vi "Main.vi"(8 "error in":errorcluster, 11 "Modbus PLC in":refnum<class "Modbus PLC.lvclass">) -> (0 "error out":errorcluster, 3 "Modbus PLC out":refnum<class "Modbus PLC.lvclass">)   [LabVIEW 2023, in "Modbus PLC.lvlib" / "Modbus PLC.lvclass"]
doc: "The <b>Queued Message Handler</b> of the Worker that owns this VI."
uses:
  Modbus PLC.lvclass
  J:/Work/Cortech/KTM 1001/Workers Hardware/Workers/Base Classes/Base Hardware/Base Hardware.lvclass
  C:/Program Files/National Instruments/LabVIEW 2023/vi.lib/addons/_Workers/Library/Classes/Worker/Worker.lvclass
  Commands.ctl
  Data.ctl
  Settings.ctl
  Workers Hardware/Workers/Base Classes/Base Hardware/rqp_Update Internal Data.ctl
  rqp_Write Rotate.ctl
  rqp_Write Termex.ctl
  rqp_Write Mix.ctl
  rqp_Write Numeric Parameter.ctl
  <vilib>/Utility/error.llb/Error Cluster From Error Code.vi
  <vilib>/ErrorRing/Error Ring.xnode
  <vilib>/addons/_Workers/Library/Classes/Message Queue/Message Queue.lvclass
  Workers Hardware/Workers/Base Classes/Base Hardware/Base Hardware.lvclass
panel:
  in  "Settings":T1={"IP Address"="localhost", "Port"=502}
  in  "Connect Btn":bool
  out "IND":T2 {"Rotate_IND" items=["стоп", "Качалка Режим Авто", "Качалка Режим Ручной"]; "Termex_IND" items=["Термостат старт"=1, "Термостат стоп"=0]; "Mix_IND" items=["Мешалка движение вперёд"=1, "Мешалка движение назад"=2, "Мешалка стоп"=0]}
  in  "CMD":T3 {"Mix_CMD" items=["Мешалка движение вперёд"=1, "Мешалка движение назад"=2, "Мешалка стоп"=9]; "Termex_CMD" items=["Термостат старт"=1, "Термостат стоп"=9]; "Rotate_CMD" items=["Качалка Дом"=1, "Качалка Режим Авто - Старт"=2, "Качалка Режим Ручной - Старт"=3, "Качалка Стоп"=9]}
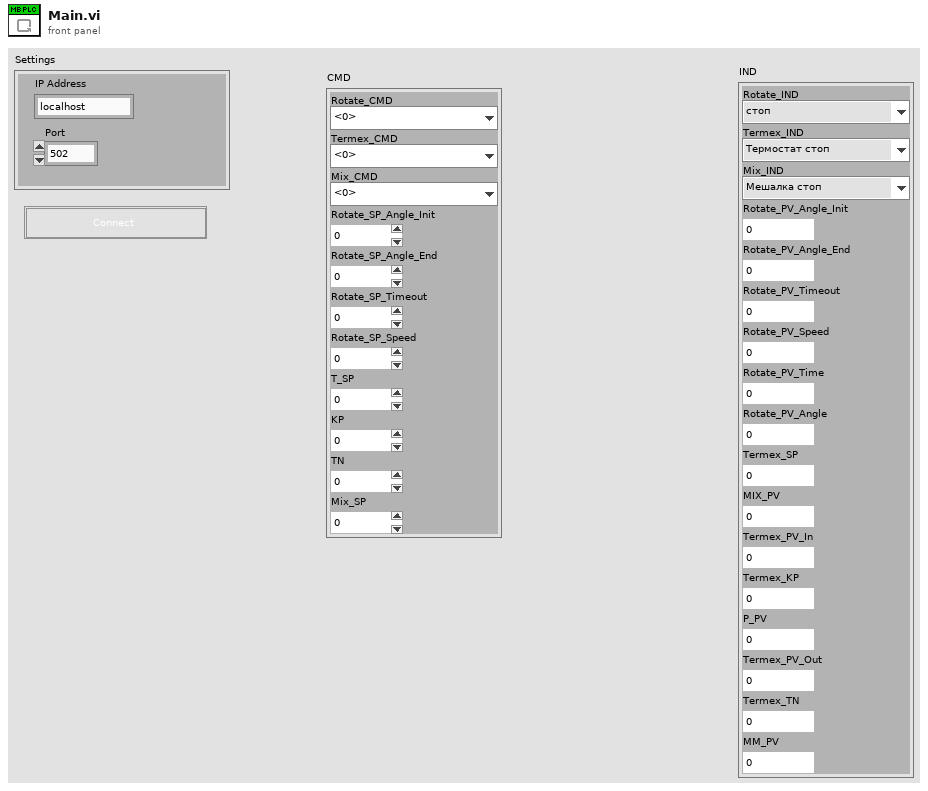
[diagram p1: front panel]
types:
  T1 = typedef "Modbus PLC.lvlib/Modbus PLC.lvclass/Settings.ctl" = cluster{"IP Address":string, "Port":u16}
  T2 = typedef "Modbus PLC.lvlib/Modbus PLC.lvclass/Data.ctl" = cluster{"Rotate_IND":u16, "Termex_IND":u16, "Mix_IND":u16, "Rotate_PV_Angle_Init":u16, "Rotate_PV_Angle_End":u16, "Rotate_PV_Timeout":u16, "Rotate_PV_Speed":u16, "Rotate_PV_Time":u16, "Rotate_PV_Angle":u16, "Termex_SP":sgl, "MIX_PV":u16, "Termex_PV_In":sgl, "Termex_KP":sgl, "P_PV":sgl, "Termex_PV_Out":sgl, "Termex_TN":sgl, "MM_PV":sgl}
  T3 = typedef "Modbus PLC.lvlib/Modbus PLC.lvclass/Commands.ctl" = cluster{"Rotate_CMD":u16, "Termex_CMD":u16, "Mix_CMD":u16, "Rotate_SP_Angle_Init":u16, "Rotate_SP_Angle_End":u16, "Rotate_SP_Timeout":u16, "Rotate_SP_Speed":u16, "T_SP":sgl, "KP":sgl, "TN":sgl, "Mix_SP":u16}
  T4 = typedef "Abstract Hardware.lvlib/Base Hardware.lvclass/rqp_Update Internal Data.ctl" = variant
  T5 = typedef "Modbus PLC.lvlib/Modbus PLC.lvclass/rqp_Write Numeric Parameter.ctl" = cluster{"Parameter":string, "Data":variant}
  T6 = typedef "Modbus PLC.lvlib/Modbus PLC.lvclass/rqp_Write Rotate.ctl" = u16
  T7 = typedef "Modbus PLC.lvlib/Modbus PLC.lvclass/rqp_Write Termex.ctl" = u16
  T8 = typedef "Modbus PLC.lvlib/Modbus PLC.lvclass/rqp_Write Mix.ctl" = u16
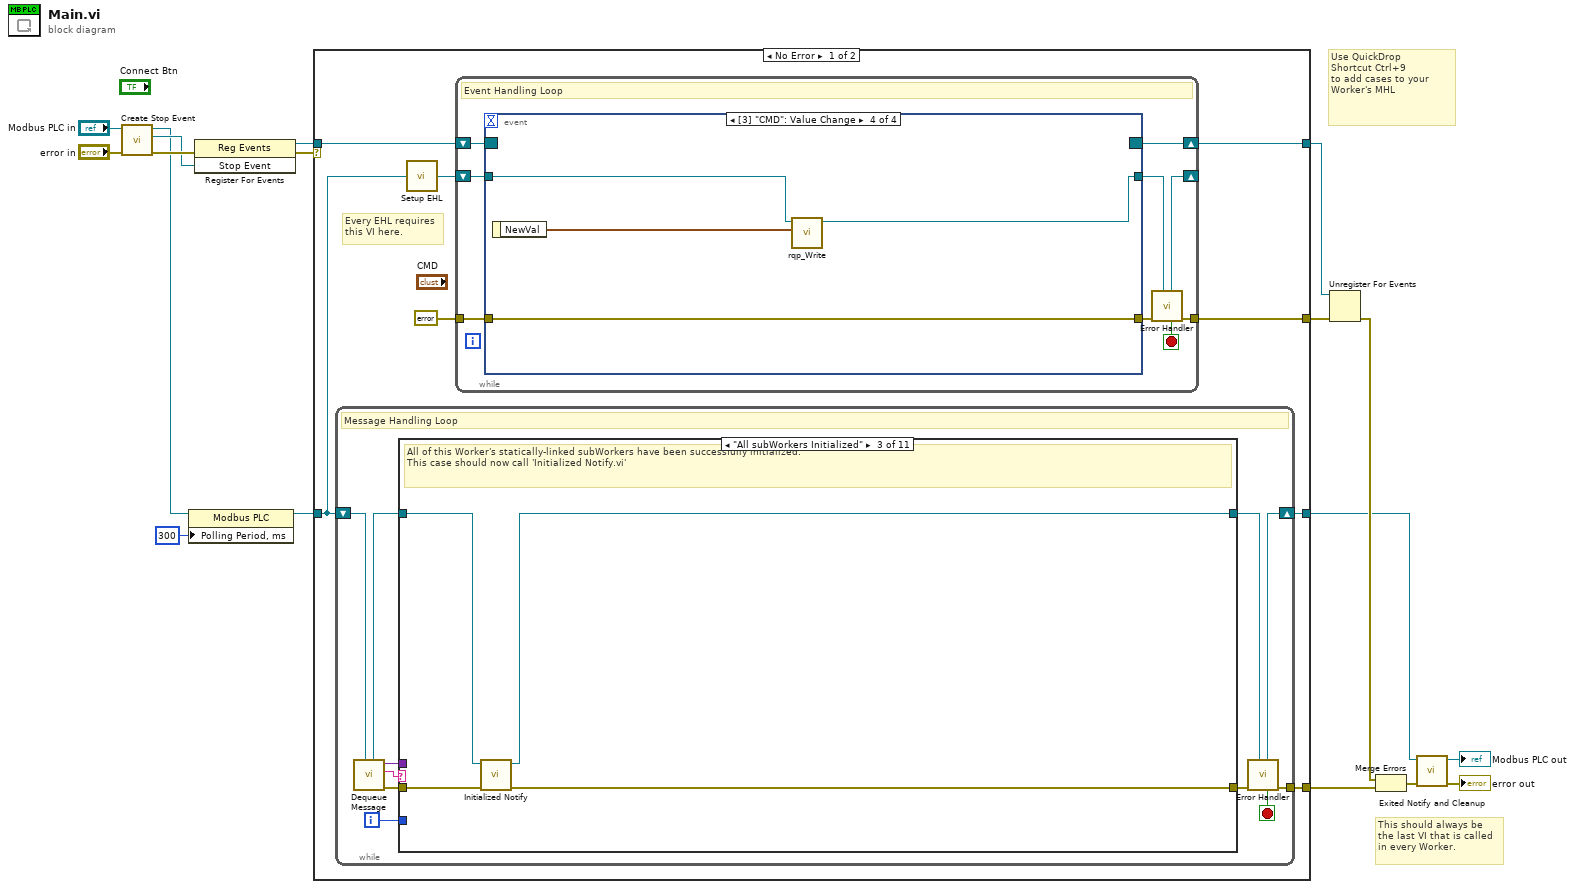
[diagram p0: block diagram]
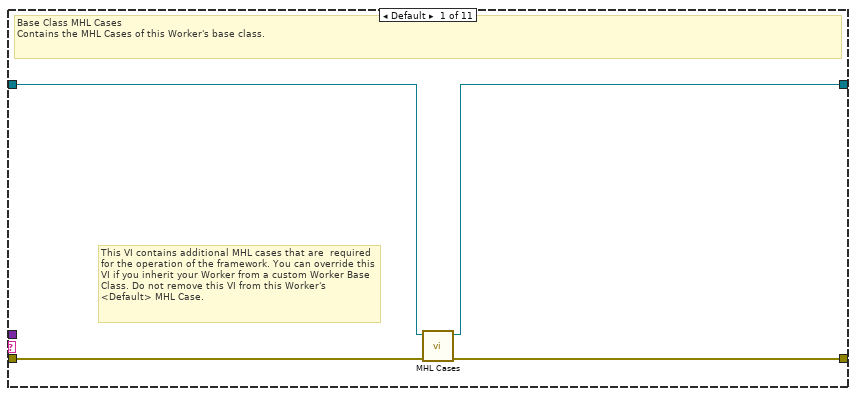
[diagram p2: hidden frame]
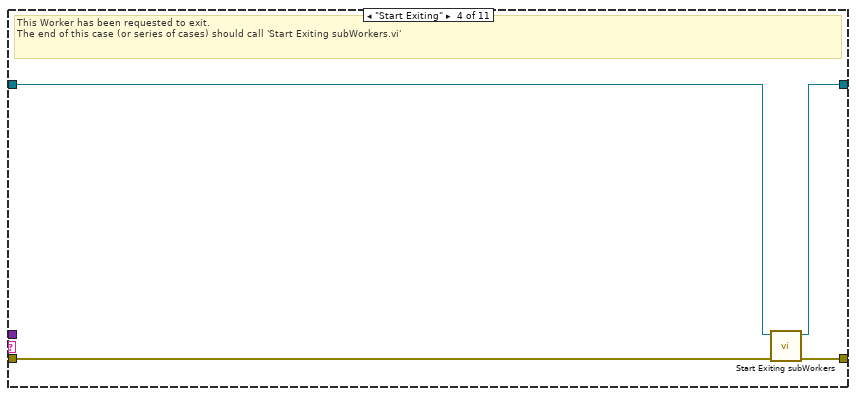
[diagram p4: hidden frame]
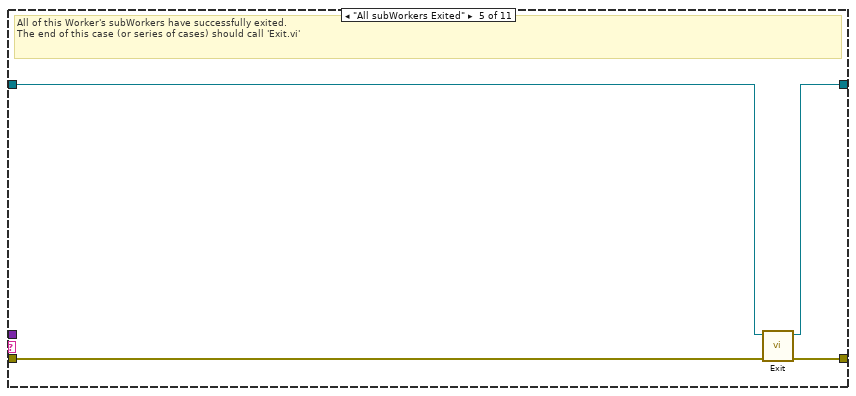
[diagram p5: hidden frame]
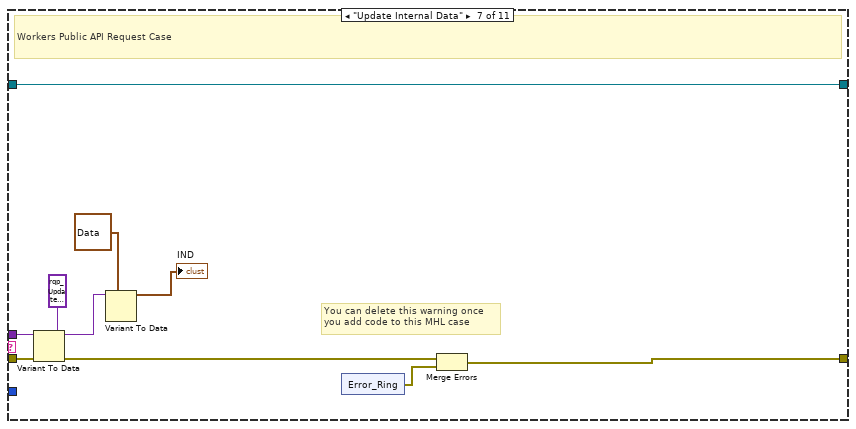
[diagram p7: hidden frame]
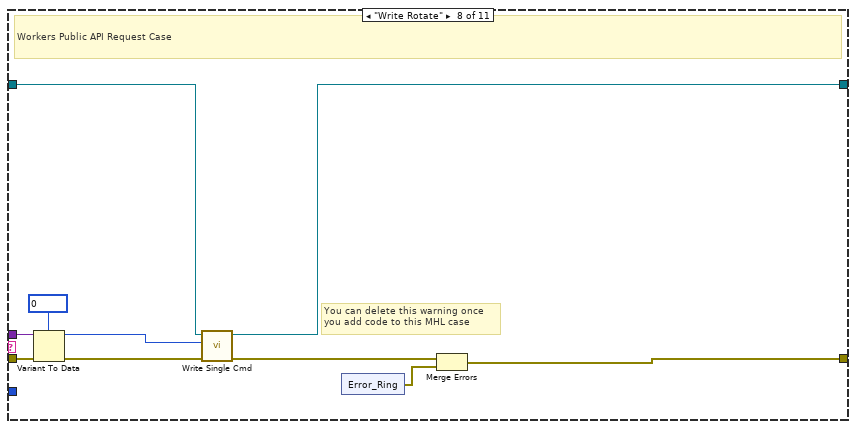
[diagram p8: hidden frame]
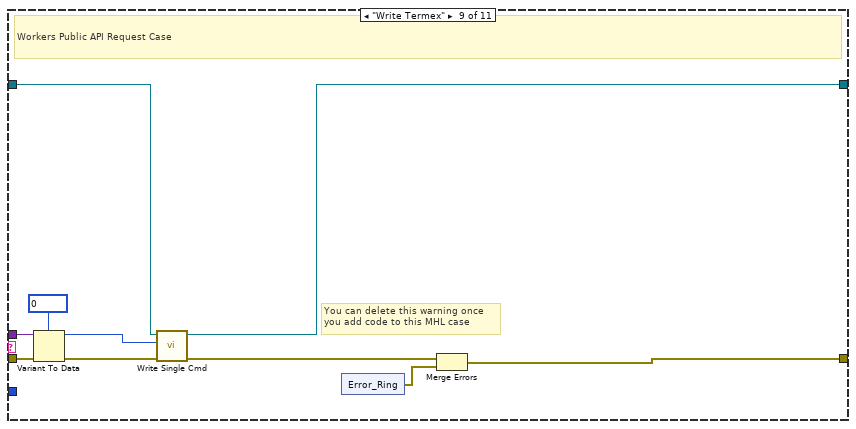
[diagram p9: hidden frame]
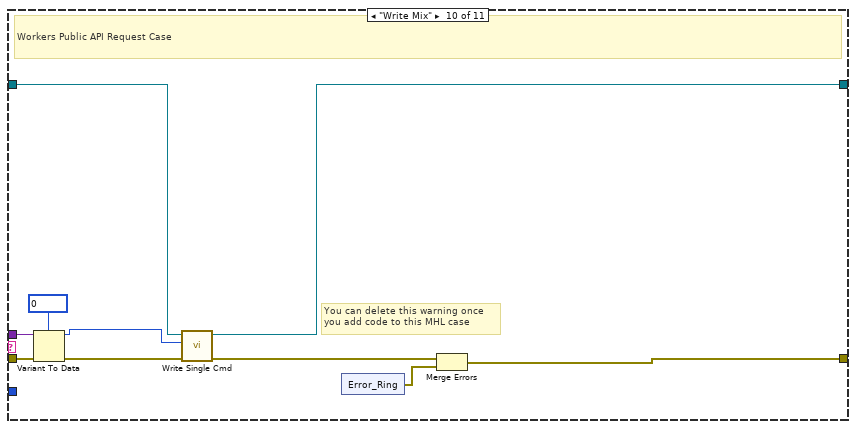
[diagram p10: hidden frame]
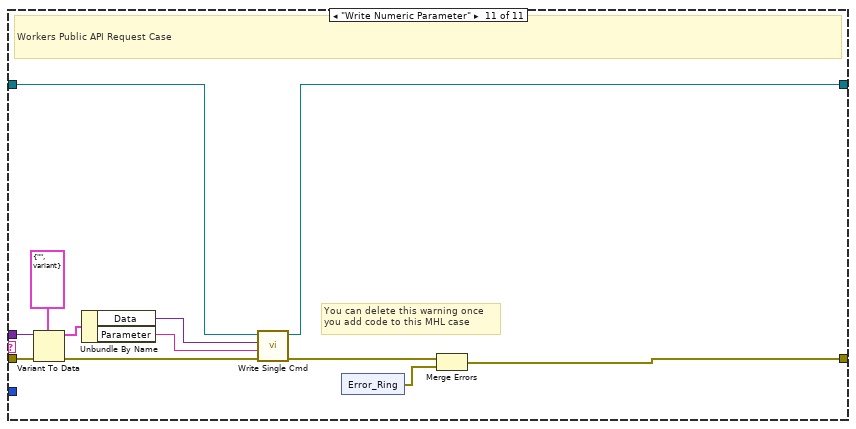
[diagram p11: hidden frame]
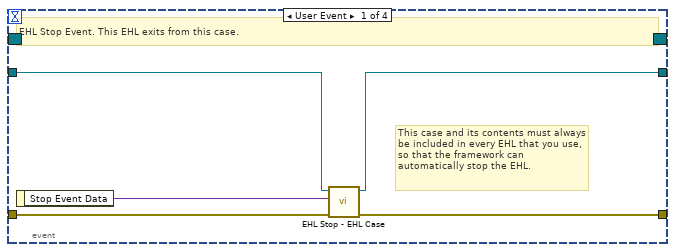
[diagram p12: hidden frame]
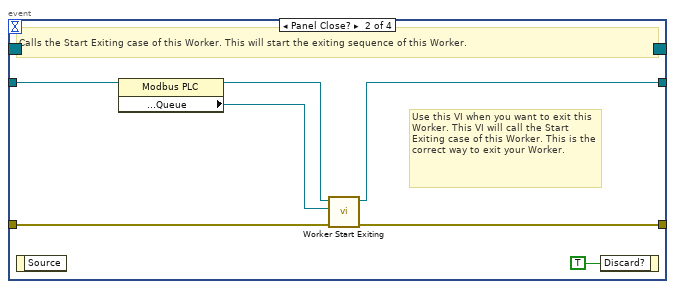
[diagram p13: hidden frame]
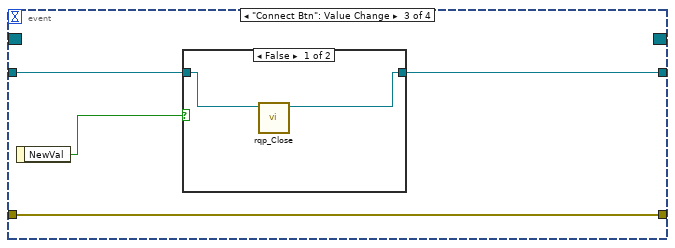
[diagram p14: hidden frame]
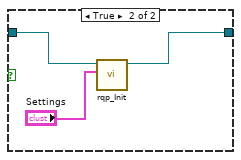
[diagram p15: hidden frame]
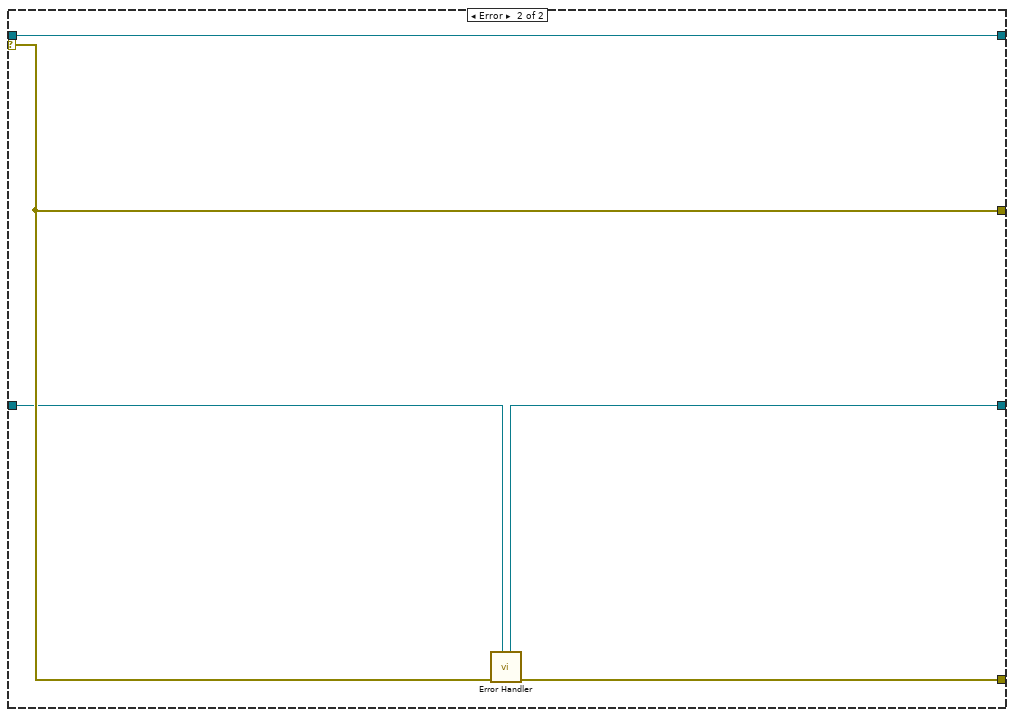
[diagram p16: hidden frame]
diagram:
  # "Use QuickDrop\nShortcut Ctrl+9\nto add cases to your\nWorker's MHL"
  # "This should always be the last VI that is called in every Worker."
  n1 = call-dynamic "Create Stop Event.vi"("error in"="error in", "Worker"="Modbus PLC in") -> ("error out"=w12:errorcluster, "Stop Event"=w9:refnum<user-event>, "Worker out"=w3:refnum<class "Modbus PLC.lvclass">)  [unwired: 7 in]
  n2 = property class="Modbus PLC"(reference=w3, "Polling Period, ms"=i64 300) -> (reference out=w2:refnum<class "Modbus PLC.lvclass">)  [unwired: 1 in, 1 out]
  n3 = register-events(error in=w12, w9) -> (reference out=w11:refnum<event-registration>, error out=w4:errorcluster)  [unwired: 1 in]
  n4 = case shown="No Error" w4 {
    tunnel: w2 -> [w20 w169]
    tunnel: [w18 w170] -> w10
    tunnel: w11 -> [w25 w171]
    tunnel: [w22 w172] -> w16
    tunnel: [w24 w171] -> w15
    tunnel: [w19 w168] -> w13
    selector: w4 -> [_ w172]
    frame No Error {
      # "Every EHL requires\nthis VI here."
      n5 = while {
        shift-right: [w34] -> w19
        shift-left: w20 -> [w36]
        tunnel: [w35] -> w18
        i -> [w27]
        stop <- w28 stop-if-true
        # "Message Handling Loop"
        n6 = call-dynamic "Dequeue Message.vi"("Worker"=w36) -> ("error out"=w33:errorcluster, "Case out"=w29:string, "Data out"=w26:variant, "Worker out"=w31:refnum<class "Modbus PLC.lvclass">)  [unwired: 6 in, 1 out]
        n7 = case "Worker MHL Case Structure (DO NOT CHANGE LABEL NAME)" shown="\"All subWorkers Initialized\"" w29 {
          tunnel: w33 -> [w40 w41 w44 w47 w54 w56 w65 w81 w96 w111 w128]
          tunnel: [w39 w41 w43 w50 w53 w56 w61 w78 w93 w108 w124] -> w32
          tunnel: w31 -> [w38 w42 w46 w48 w52 w55 w66 w73 w89 w103 w119]
          tunnel: [w37 w42 w45 w49 w51 w55 w66 w72 w88 w104 w120] -> w30
          tunnel: w27 -> [_ _ _ _ _ _ _ _ _ _ _]
          tunnel: w26 -> [_ _ _ _ _ _ w62 w79 w94 w109 w126]
          frame Default {
            # "This VI contains additional MHL cases that are  required for the operation of the framework. You can override this VI if you inherit your Worker from a custom Worker Base Class. Do not remove this VI from this Worker's <Default> MHL Case."
            # "Base Class MHL Cases\nContains the MHL Cases of this Worker's base class."
            n8 = call-dynamic "MHL Cases.vi"("error in"=w40, "Base Hardware in"=w38) -> ("error out"=w39:errorcluster, "Base Hardware out"=w37:refnum<class "Modbus PLC.lvclass">)  [unwired: 8 in]
          }
          frame "------------ FRAMEWORK CASES -----------" {
            # "Start of Workers Framework Cases"
          }
          frame "All subWorkers Initialized" {
            # "All of this Worker's statically-linked subWorkers have been successfully initialized.\nThis case should now call 'Initialized Notify.vi'"
            n9 = call-dynamic "Initialized Notify.vi"("error in"=w44, "Worker"=w46) -> ("error out"=w43:errorcluster, "dup Worker out"=w45:refnum<class "Modbus PLC.lvclass">)  [unwired: 8 in]
          }
          frame "Start Exiting" {
            # "This Worker has been requested to exit. \nThe end of this case (or series of cases) should call 'Start Exiting subWorkers.vi'"
            n10 = call-dynamic "Start Exiting subWorkers.vi"("error_in"=w47, "Worker"=w48) -> ("error out"=w50:errorcluster, "dup Worker out"=w49:refnum<class "Modbus PLC.lvclass">)  [unwired: 8 in]
          }
          frame "All subWorkers Exited" {
            # "All of this Worker's subWorkers have successfully exited. \nThe end of this case (or series of cases) should call 'Exit.vi'"
            n11 = call-dynamic "Exit.vi"("error_in"=w54, "Worker"=w52) -> ("error out"=w53:errorcluster, "dup Worker out"=w51:refnum<class "Modbus PLC.lvclass">)  [unwired: 8 in]
          }
          frame "------------- PUBLIC API CASES -------------" {
            # "Start of Workers Public API Cases"
          }
          frame "Update Internal Data" {
            # "You can delete this warning once\nyou add code to this MHL case"
            # "Workers Public API Request Case"
            n12 = Variant To Data(error in=w65, type=T4 variant(string "") ("Data"), Variant=w62) -> (data=w59:T4, error out=w64:errorcluster)
            n13 = Variant To Data(type=T2 {"Rotate_IND"=0, "Termex_IND"=0, "Mix_IND"=0, "Rotate_PV_Angle_Init"=0, "Rotate_PV_Angle_End"=0, "Rotate_PV_Timeout"=0, "Rotate_PV_Speed"=0, "Rotate_PV_Time"=0, "Rotate_PV_Angle"=0, "Termex_SP"=0.0, "MIX_PV"=0, "Termex_PV_In"=0.0, "Termex_KP"=0.0, "P_PV"=0.0, "Termex_PV_Out"=0.0, "Termex_TN"=0.0, "MM_PV"=0.0} ("IND"), Variant=w59) -> (data=→"IND":T2)  [unwired: 1 in, 1 out]
            n14 = xnode ("Error_Ring")() -> ("error out"=w60:errorcluster)
            n15 = Merge Errors(w64, w60) -> (w61:errorcluster)
          }
          frame "Write Rotate" {
            w80 = T6 0 items=["Качалка Дом"=1, "Качалка Режим Авто - Старт"=2, "Качалка Режим Ручной - Старт"=3, "Качалка Стоп"=9] ("Data")
            # "You can delete this warning once\nyou add code to this MHL case"
            # "Workers Public API Request Case"
            n16 = Variant To Data(error in=w81, type=w80, Variant=w79) -> (data=w74:T6, error out=w76:errorcluster)
            n17 = call "Write Single Cmd.vi"("error in (no error)"=w76, "variant"=w74, "Modbus PLC in"=w73) -> ("error out"=w75:errorcluster, "Modbus PLC out"=w72:refnum<class "Modbus PLC.lvclass">)  [unwired: 7 in]
            n18 = xnode ("Error_Ring")() -> ("error out"=w77:errorcluster)
            n19 = Merge Errors(w75, w77) -> (w78:errorcluster)
          }
          frame "Write Termex" {
            w95 = T7 0 items=["Термостат старт"=1, "Термостат стоп"=9] ("Data")
            # "You can delete this warning once\nyou add code to this MHL case"
            # "Workers Public API Request Case"
            n20 = Variant To Data(error in=w96, type=w95, Variant=w94) -> (data=w90:T7, error out=w91:errorcluster)
            n21 = call "Write Single Cmd.vi"("error in (no error)"=w91, "variant"=w90, "Modbus PLC in"=w89) -> ("error out"=w87:errorcluster, "Modbus PLC out"=w88:refnum<class "Modbus PLC.lvclass">)  [unwired: 7 in]
            n22 = xnode ("Error_Ring")() -> ("error out"=w92:errorcluster)
            n23 = Merge Errors(w87, w92) -> (w93:errorcluster)
          }
          frame "Write Mix" {
            w110 = T8 0 items=["Мешалка движение вперёд"=1, "Мешалка движение назад"=2, "Мешалка стоп"=9] ("Data")
            # "You can delete this warning once\nyou add code to this MHL case"
            # "Workers Public API Request Case"
            n24 = Variant To Data(error in=w111, type=w110, Variant=w109) -> (data=w102:T8, error out=w106:errorcluster)
            n25 = call "Write Single Cmd.vi"("error in (no error)"=w106, "variant"=w102, "Modbus PLC in"=w103) -> ("error out"=w105:errorcluster, "Modbus PLC out"=w104:refnum<class "Modbus PLC.lvclass">)  [unwired: 7 in]
            n26 = xnode ("Error_Ring")() -> ("error out"=w107:errorcluster)
            n27 = Merge Errors(w105, w107) -> (w108:errorcluster)
          }
          frame "Write Numeric Parameter" {
            # "You can delete this warning once\nyou add code to this MHL case"
            # "Workers Public API Request Case"
            n28 = Variant To Data(error in=w128, type=T5 {"Parameter"="", "Data"=variant(string "")} ("Data"), Variant=w126) -> (data=w125:T5, error out=w122:errorcluster)
            n29 = Unbundle By Name(w125) -> ("Data"=w117:variant, "Parameter"=w118:string)
            n30 = call "Write Single Cmd.vi"("error in (no error)"=w122, "Name"=w118, "variant"=w117, "Modbus PLC in"=w119) -> ("error out"=w121:errorcluster, "Modbus PLC out"=w120:refnum<class "Modbus PLC.lvclass">)  [unwired: 6 in]
            n31 = xnode ("Error_Ring")() -> ("error out"=w123:errorcluster)
            n32 = Merge Errors(w121, w123) -> (w124:errorcluster)
          }
        }
        n33 = call-dynamic "Error Handler.vi"("Worker"=w30, "error_in"=w32) -> ("error out"=w35:errorcluster, "Stop Loop"=w28:bool, "Worker out"=w34:refnum<class "Modbus PLC.lvclass">)  [unwired: 7 in]
      }
      n34 = call-dynamic "Setup EHL.vi"("Worker"=w20) -> ("Worker out"=w21:refnum<class "Modbus PLC.lvclass">)  [unwired: 14 in]
      n35 = while "Event Handling Loop" {
        shift-right: [w142] -> w24
        shift-left: w25 -> [w141]
        tunnel: [w137] -> w22
        tunnel: errorcluster {"status"=FALSE, "code"=0, "source"=""} ("error constant") -> [w139]
        shift-right: [w135] -> _
        shift-left: w21 -> [w140]
        stop <- w134 stop-if-true
        # "Event Handling Loop"
        n36 = event shown="[3] \"CMD\": Value Change" {
          selector: w141 -> [_ _ _ _]
          dyn-events: [_ _ _ _] -> w142
          timeout: _ -> [_ _ _ _]
          tunnel: [w146 w153 w158 w167] -> w138
          tunnel: w139 -> [w147 w152 w158 w167]
          tunnel: w140 -> [w145 w151 w156 w166]
          tunnel: [w144 w150 w155 w165] -> w136
          event User Event {
            # "This case and its contents must always be included in every EHL that you use, so that the framework can automatically stop the EHL."
            # "EHL Stop Event. This EHL exits from this case."
            n37 = event-data() -> ("Stop Event Data"=w143:variant)  [unwired: 1 in]
            n38 = call-dynamic "EHL Stop - EHL Case.vi"("error in"=w147, "Stop Event Data"=w143, "Worker"=w145) -> ("error out"=w146:errorcluster, "Worker out"=w144:refnum<class "Modbus PLC.lvclass">)  [unwired: 7 in]
          }
          event Panel Close? {
            # "Use this VI when you want to exit this Worker. This VI will call the Start Exiting case of this Worker. This is the correct way to exit your Worker."
            # "Calls the Start Exiting case of this Worker. This will start the exiting sequence of this Worker."
            n39 = event-data() -> ()  [unwired: 1 in, 1 out]
            n40 = property class="Modbus PLC"(reference=w151) -> (reference out=w149:refnum<class "Modbus PLC.lvclass">, "Accessors:Read:Public API:Queue"=w148:refnum<class "Message Queue.lvclass">)  [unwired: 1 in, 1 out]
            n41 = call-dynamic "Worker Start Exiting.vi"("error_in"=w152, "Message Queue"=w148, "Worker"=w149) -> ("error out"=w153:errorcluster, "dup Worker out"=w150:refnum<class "Modbus PLC.lvclass">)  [unwired: 7 in]
            n42 = event-data("Discard?"=TRUE) -> ()  [unwired: 1 in, 1 out]
          }
          event "Connect Btn": Value Change {
            n43 = event-data() -> ("NewVal"=w157:bool)  [unwired: 1 in]
            n44 = case shown="False" w157 {
              tunnel: w156 -> [w160 w163]
              tunnel: [w159 w162] -> w155
              frame False {
                n45 = call-dynamic "rqp_Close.vi"("Base Hardware in"=w160) -> ("dup Base Hardware out"=w159:refnum<class "Modbus PLC.lvclass">)  [unwired: 9 in, 1 out]
              }
              frame True {
                n46 = call-dynamic "rqp_Init.vi"("Data in"="Settings", "Base Hardware in"=w163) -> ("dup Base Hardware out"=w162:refnum<class "Modbus PLC.lvclass">)  [unwired: 8 in, 1 out]
              }
            }
          }
          event Value Change {
            n47 = event-data() -> ("NewVal"=w164:T3)  [unwired: 1 in]
            n48 = call-dynamic "rqp_Write.vi"("Data in"=w164, "Base Hardware in"=w166) -> ("dup Base Hardware out"=w165:refnum<class "Modbus PLC.lvclass">)  [unwired: 8 in, 1 out]
          }
        }
        n49 = call-dynamic "Error Handler.vi"("Worker"=w136, "error_in"=w138) -> ("error out"=w137:errorcluster, "Stop Loop"=w134:bool, "Worker out"=w135:refnum<class "Modbus PLC.lvclass">)  [unwired: 7 in]
      }
    }
    frame Error {
      n50 = call-dynamic "Error Handler.vi"("Worker"=w169, "error_in"=w172) -> ("error out"=w170:errorcluster, "Worker out"=w168:refnum<class "Modbus PLC.lvclass">)  [unwired: 7 in, 1 out]
    }
  }
  n51 = Unregister For Events(event registration refnum=w15, error in=w16) -> (error out=w17:errorcluster)
  n52 = Merge Errors(w17, w10) -> (w14:errorcluster)
  n53 = call-dynamic "Exited Notify and Cleanup.vi"("error_in"=w14, "Worker"=w13) -> ("error out"=→"error out":errorcluster, "dup Worker out"=→"Modbus PLC out":refnum<class "Modbus PLC.lvclass">)  [unwired: 8 in]
